vi "Measure Output.vi"(8 "error in":errorcluster, 11 "69X_79X in":refnum<class "69X_79X.lvclass">) -> (0 "error out":errorcluster, 1 "Current":dbl[](array[numeric]), 2 "Voltage":dbl[](array[numeric]), 3 "69X_79X out":refnum<class "69X_79X.lvclass">)   [LabVIEW 2019, in "69X_79X.lvlib" / "69X_79X.lvclass"]
uses:
  Library/69X_79X.lvclass
  Library/69X_79X.lvclass/69X_79X.ctl
  <instrlib>/Agilent N6900 N7900 Series/Agilent N6900 N7900 Series.lvlib
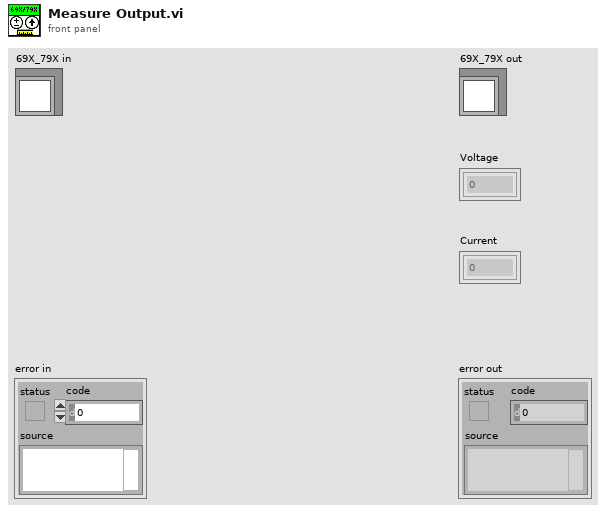
[diagram p1: front panel]
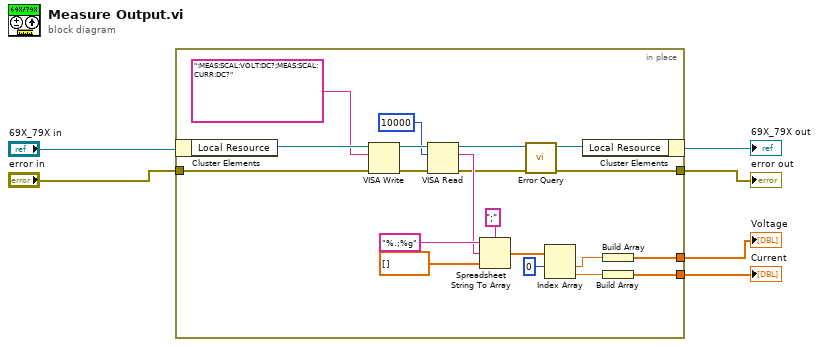
[diagram p0: block diagram]
diagram:
  n1 = in-place {
    in-place-border: "error in" -> [w14]
    in-place-border: [w13] -> w3
    in-place-border: [w8] -> w2
    in-place-border: [w7] -> w1
    n2 = in-place-cluster #1("69X_79X in") -> ("Local Resource"=w26:refnum<visa-resource-name>)
    n3 = VISA Write(VISA resource name=w26, write buffer=":MEAS:SCAL:VOLT:DC?;MEAS:SCAL:CURR:DC?", error in (no error)=w14) -> (VISA resource name out=w23:refnum<visa-resource-name>, error out=w24:errorcluster)  [unwired: 1 out]
    n4 = VISA Read(VISA resource name=w23, byte count=u32 10000, error in (no error)=w24) -> (VISA resource name out=w17:refnum<visa-resource-name>, read buffer=w19:string, error out=w16:errorcluster)  [unwired: 1 out]
    n5 = Spreadsheet String To Array(delimiter (Tab)=";", format string="%.;%g", spreadsheet string=w19, array type (2D Dbl)=dbl[] []) -> (array=w12:dbl[])
    n6 = call <instrlib>:"Error Query.vi"("error in (no error)"=w16, "VISA resource name"=w17) -> ("error out"=w13:errorcluster, "VISA resource name out"=w15:refnum<visa-resource-name>)  [unwired: 6 in, 2 out]
    n7 = Index Array(array=w12, index #1=0 ("index")) -> (element #1=w10:dbl, element #2=w9:dbl)  [unwired: 1 in]
    n8 = in-place-cluster #1("Local Resource"=w15) -> (→"69X_79X out":refnum<class "69X_79X.lvclass">)
    n9 = Build Array(w10) -> (w8:dbl[])
    n10 = Build Array(w9) -> (w7:dbl[])
  }
  "error out" <- w3
  "Current" <- w1
  "Voltage" <- w2
